vi "run.vi"(6 "deviceDatabase":refnum<class "deviceDataBase.lvclass">, 7 "HardwareList out":refnum<class "HWConfiguration.lvclass">, 8 "error in (no error)":errorcluster, 9 "debuggingFlag":bool, 10 "HWControllerEvents":refnum<class "HWControllerEvents.lvclass">, 11 "HWController in":refnum<class "HWController.lvclass">) -> (0 "error out":errorcluster, 2 "HWControllerEvents out":refnum<class "HWControllerEvents.lvclass">, 3 "HWController out":refnum<class "HWController.lvclass">)   [LabVIEW 2009, in "Hardware.lvlib" / "HWControllers.lvlib" / "HWController.lvclass"]
doc: "HWController run.\n\nThis starts the Hardware Controller who is responsible for manipulating the hardware, and running the compilers."
uses:
  HWController.lvclass
  HWControllerEvents/HWControllerEvents.lvclass
  Tools/DatabaseHelpers/DbConnection/DeviceDataBase/deviceDataBase.lvclass
  HardwareConfiguration/HWConfiguration.lvclass
  HWController.lvclass/HWController.ctl
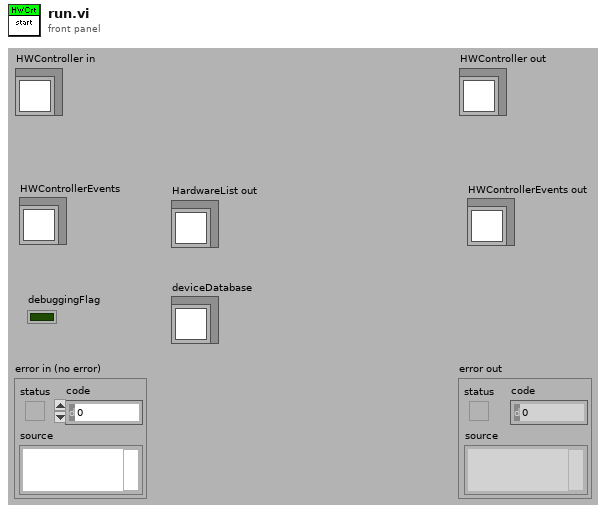
[diagram p1: front panel]
types:
  T1 = enum16{"Ready", "Compiling", "Configured", "Running", "Stopping", "Unresolved Error"}
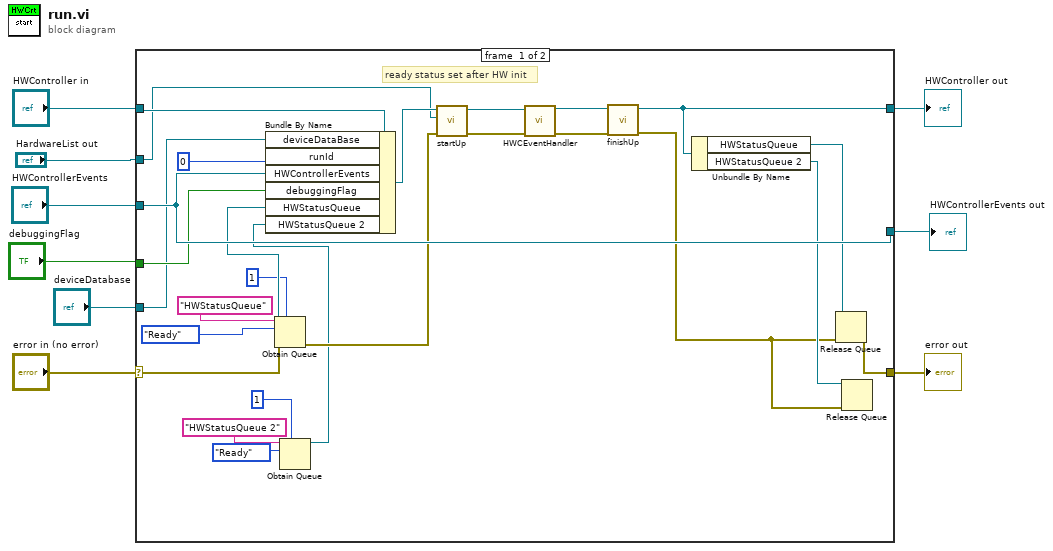
[diagram p0: block diagram]
diagram:
  n1 = case shown="No Error" "error in (no error)" {
    selector: "error in (no error)" -> [w24 w37]
    tunnel: [w17 w37] -> w8
    tunnel: [w19 w36] -> w6
    tunnel: "HWController in" -> [w31 w36]
    tunnel: "HWControllerEvents" -> [w29 _]
    tunnel: [w29 _] -> w4
    tunnel: "debuggingFlag" -> [w28 _]
    tunnel: "deviceDatabase" -> [w26 _]
    tunnel: "HardwareList out" -> [w25 _]
    frame #0 {
      # "ready status set after HW init"
      n2 = Obtain Queue(max queue size (-1, unlimited)=1, name (unnamed)="HWStatusQueue", element data type=T1."Ready" ("status"), error in (no error)=w24) -> (queue out=w20:refnum<queue>, error out=w23:errorcluster)  [unwired: 1 in, 1 out]
      n3 = Obtain Queue(max queue size (-1, unlimited)=1, name (unnamed)="HWStatusQueue 2", element data type=T1."Ready" ("status")) -> (queue out=w12:refnum<queue>)  [unwired: 2 in, 2 out]
      n4 = Bundle By Name(cluster=w31, "deviceDataBase"=w26, "runId"=0, "HWControllerEvents"=w29, "debuggingFlag"=w28, "HWStatusQueue"=w20, "HWStatusQueue 2"=w12) -> (w30:refnum<class "HWController.lvclass">)
      n5 = call-dynamic "startUp.vi"("error in (no error)"=w23, "HardwareList out"=w25, "HWController in"=w30) -> ("error out"=w35:errorcluster, "HWController out"=w34:refnum<class "HWController.lvclass">)  [unwired: 7 in]
      n6 = call-dynamic "HWCEventHandler.vi"("error in (no error)"=w35, "HWController in"=w34) -> ("error out"=w33:errorcluster, "HWController out"=w32:refnum<class "HWController.lvclass">)  [unwired: 8 in]
      n7 = call-dynamic "finishUp.vi"("error in (no error)"=w33, "HWController in"=w32) -> ("error out"=w10:errorcluster, "HWController out"=w19:refnum<class "HWController.lvclass">)  [unwired: 8 in]
      n8 = Unbundle By Name(w19) -> ("HWStatusQueue"=w18:refnum<queue>, "HWStatusQueue 2"=w11:refnum<queue>)
      n9 = Release Queue(queue=w18, error in (no error)=w10) -> (error out=w17:errorcluster)  [unwired: 1 in, 2 out]
      n10 = Release Queue(queue=w11, error in (no error)=w10) -> ()  [unwired: 1 in, 3 out]
    }
    frame #1 {
    }
  }
  "error out" <- w8
  "HWController out" <- w6
  "HWControllerEvents out" <- w4
